vi "Accelerometer.vi"(11 "Queue ref":T1) -> ()   [LabVIEW 2022 SP3]
uses:
  Controls/All Queue.ctl
  Controls/DAQ case.ctl
  Controls/UI Data.ctl
  Controls/All Loop Status.ctl
  <vilib>/DAQmx/read.llb/DAQmx Read (Analog 1D Wfm NChan NSamp).vi
  Create Task/ACC Create Task.vi
  <vilib>/DAQmx/configure/timing.llb/DAQmx Timing (Sample Clock).vi
  Sub VI's/Global 1.vi
  <vilib>/DAQmx/miscellaneous.llb/DAQmx Fill In Error Info.vi
panel:
  # "TC channel list"
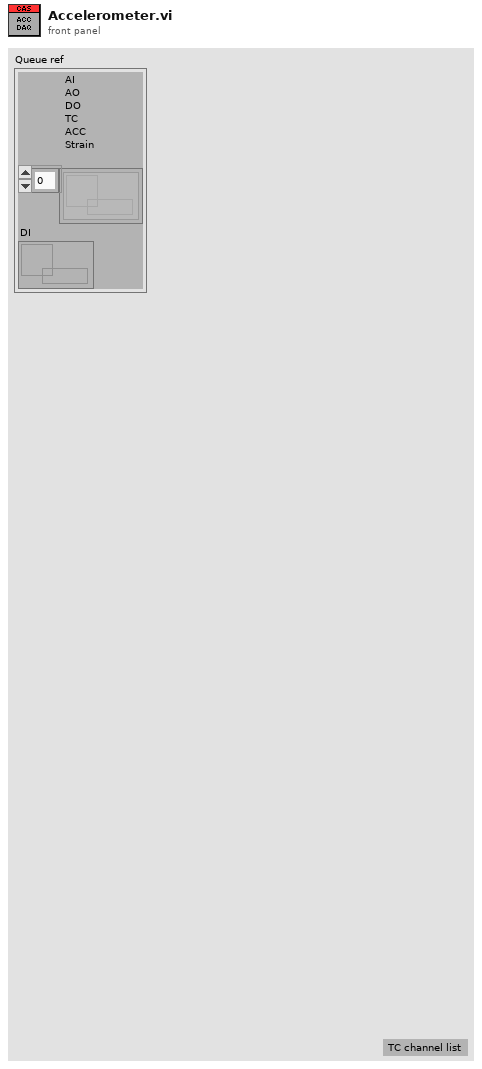
[diagram p1: front panel]
types:
  T1 = typedef "All Queue.ctl" = cluster{"AI\nAO\nDO\nTC\nACC\nStrain":refnum<queue>[], "DI":refnum<queue>}
  T2 = cluster{"in progress?":bool, "Queue ref":T1, "Start DAQ":refnum<notifier>, "UI Data":refnum<notifier>, "task out":refnum<k21>, "ACC Ref":refnum<queue>, "SPC":i32}
  T3 = typedef "DAQ case.ctl" = enum16{"Initailise", "Create Task", "Polevent", "Acquire", "Stop DAQ", "Error", "Exit"}
  T4 = typedef "All Loop Status.ctl" = enum16{"AI", "AO", "DI", "DO", "TC", "Strain", "ACC", "RT", "Log"}
  T5 = enum16{"Init", "Read 'All'", "Read 'n'", "Read '1'", "Write '1'", "Write 'n'", "Write 'All'"}
  T6 = typedef "All Notifer.ctl" = cluster{"UI Data":refnum<notifier>, "Start DAQ":refnum<notifier>, "Start Log":refnum<notifier>}
  T7 = cluster{"Analog input":bool, "Analog Output":bool, "Digital input":bool, "Digital output":bool, "Thermocouple":bool, "Strain Gauge":bool, "Accelerometer":bool}
  T8 = typedef "Config.ctl" = cluster{"AO config":cluster{"Channel_Name":string, "Channel_Number":string, "Default_Value":dbl, "Units":string}[], "AI config":cluster{"Channel_Name":string, "Channel_Number":string, "Pre_Scale_min":dbl, "Pre_Scale_max":dbl, "Sensor_min":dbl, "Sensor_max":dbl, "Units":string}[], "DI config":cluster{"Channel_Name":string, "Channel_Number":string, "Default_Value":bool, "DI invert?":bool}[], "DO config":cluster{"Channel_Name":string, "Channel_Number":string, "Default_Value":bool, "DO invert?":bool}[], "TC config":cluster{"Channel_Name":string, "Channel_Number":string, "Pre_Scale_min":dbl, "Pre_Scale_max":dbl, "units":i32, " type":i32}[], "ACC config":cluster{"Channel_Name":string, "Channel_Number":string, "Pre_Scale_min":dbl, "Pre_Scale_max":dbl, "Terminal configuration":i32, "Sensitivity":dbl, "Sensitivity units":i32}[], "SG config":cluster{"Channel_Name":string, "Channel_Number":string, "Pre_Scale_min":dbl, "Pre_Scale_max":dbl}[], "Strain Gauge Settings":cluster{"poisson ratio":dbl, "nominal gage resistance":dbl, "gage factor":dbl}, "bridge information":cluster{"strain configuration":i32, "lead wire resistance":dbl, "initial bridge voltage":dbl, "voltage excitation source":i32, "voltage excitation value":dbl}, "Sample Rate":cluster{"AI Sample Rate":dbl, "AO Sample Rate":dbl, "DI Sample Rate":dbl, "TC Sample Rate":dbl, "DO Sample Rate":dbl, "SG Sample Rate":dbl, "ACC Sample Rate":dbl}}
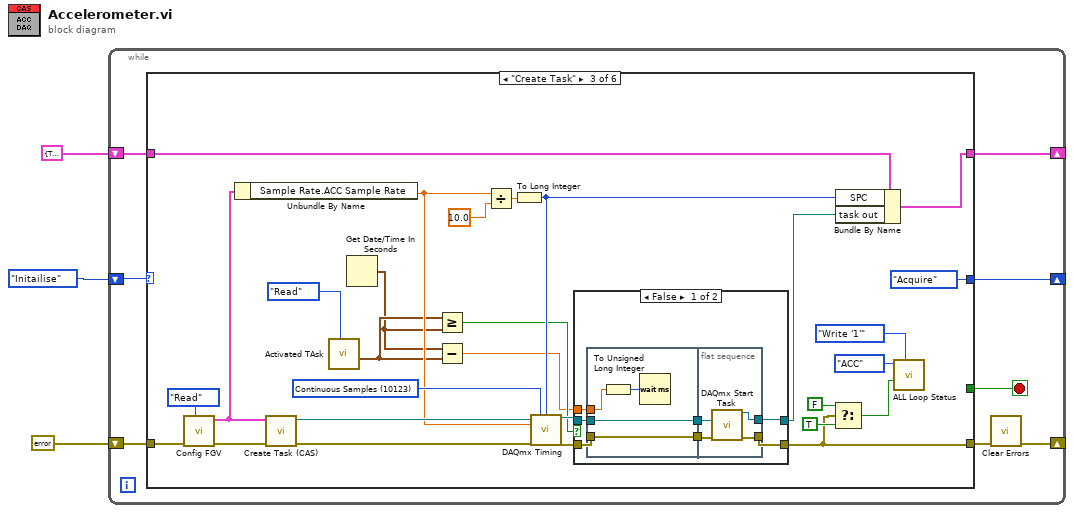
[diagram p0: block diagram]
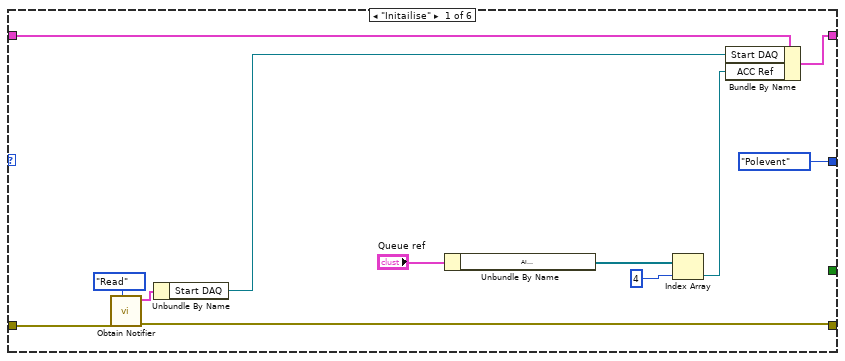
[diagram p2: hidden frame]
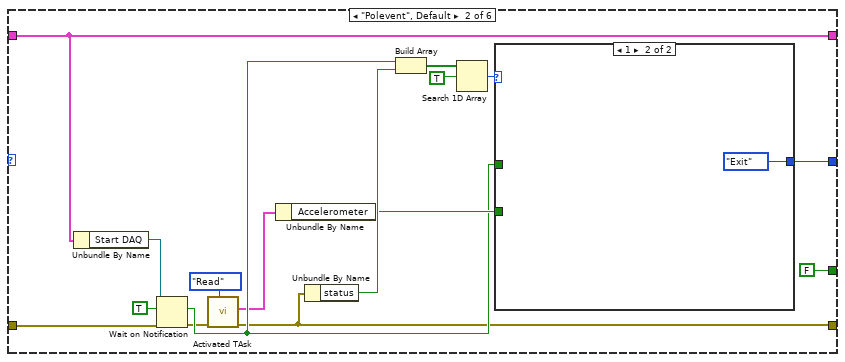
[diagram p3: hidden frame]
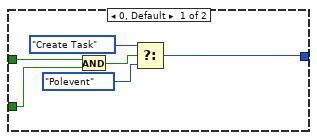
[diagram p4: hidden frame]
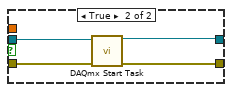
[diagram p5: hidden frame]
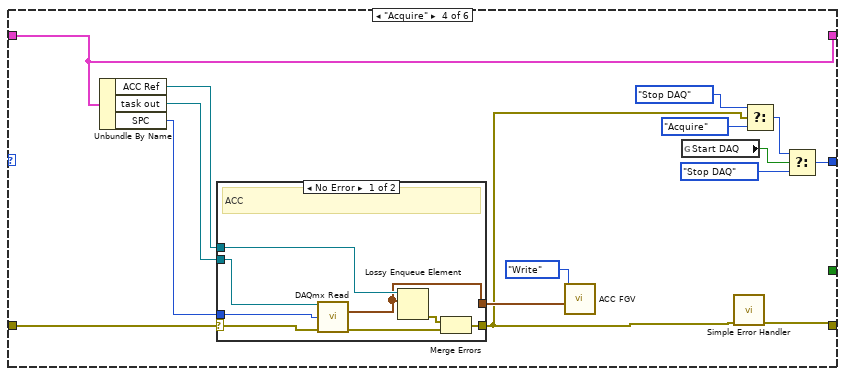
[diagram p6: hidden frame]
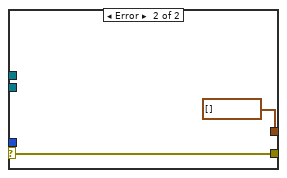
[diagram p7: hidden frame]
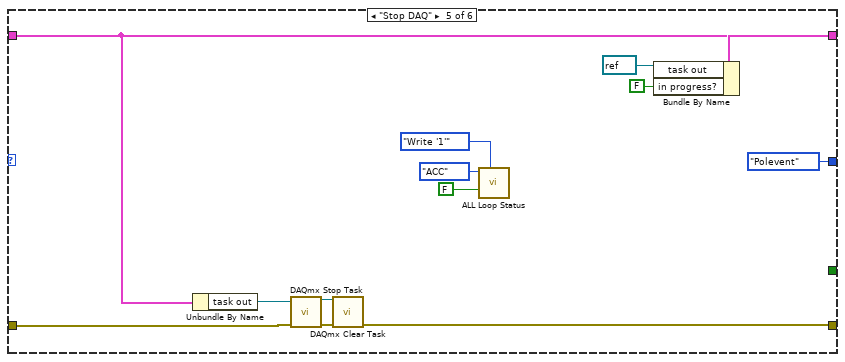
[diagram p8: hidden frame]
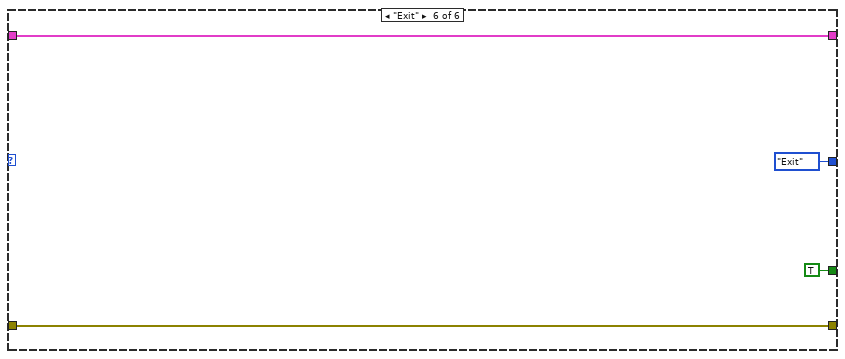
[diagram p9: hidden frame]
diagram:
  n1 = while {
    shift-right: [w4] -> _
    shift-left: errorcluster {"status"=FALSE, "code"=0, "source"=""} ("error out") -> [w10]
    shift-right: [w8] -> _
    shift-left: T2 {"in progress?"=TRUE, "Queue ref"={"AI\nAO\nDO\nTC\nACC\nStrain"=[], "DI"=refnum}, "Start DAQ"=refnum, "UI Data"=refnum, "task out"="", "ACC Ref"=refnum, "SPC"=0} -> [w9]
    shift-right: [w7] -> _
    shift-left: DAQ_case."Initailise" -> [w6]
    stop <- w11 stop-if-true
    n2 = case shown="\"Create Task\"" w6 {
      tunnel: [_ FALSE _ _ _ TRUE] -> w11
      tunnel: w10 -> [w22 w27 w71 w101 w123 w135]
      tunnel: [w21 w25 w54 w95 w124 w135] -> w5
      tunnel: w9 -> [w19 w37 w73 w102 w128 w134]
      tunnel: [w17 w37 w72 w102 w129 w134] -> w8
      tunnel: [DAQ_case."Polevent" w38 DAQ_case."Acquire" w103 DAQ_case."Polevent" DAQ_case."Exit"] -> w7
      frame "Initailise" {
        n3 = call "Obtain Notifier.vi"("Case"=enum16{"Obtain", "Read"}."Read", "error in (no error)"=w22) -> ("error out"=w21:errorcluster, "notifiers out"=w20:T6)  [unwired: 8 in]
        n4 = Unbundle By Name(w20) -> ("Start DAQ"=w18:refnum<notifier>)
        n5 = Unbundle By Name("Queue ref") -> ("AI\nAO\nDO\nTC\nACC\nStrain"=w14:refnum<queue>[])
        n6 = Index Array(array=w14, index=4) -> (element=w13:refnum<queue>)
        n7 = Bundle By Name(cluster=w19, "Start DAQ"=w18, "ACC Ref"=w13) -> (w17:T2)
      }
      frame "Polevent", Default {
        n8 = Unbundle By Name(w37) -> ("Start DAQ"=w36:refnum<notifier>)
        n9 = Wait on Notification(notifier=w36, ignore previous (F)=TRUE, error in (no error)=w27) -> (notification=w28:bool, error out=w26:errorcluster)  [unwired: 1 in, 2 out]
        n10 = call "Activated TAsk.vi"("Enum"=enum16{"Read", "Write"}."Read", "error in (no error)"=w26) -> ("error out"=w25:errorcluster, "Activate Task 2"=w24:T7)  [unwired: 7 in, 1 out]
        n11 = Unbundle By Name(w24) -> ("Accelerometer"=w29:bool)
        n12 = Unbundle By Name(w25) -> ("status"=w35:bool)
        n13 = Build Array(w28, w35) -> (w33:bool[])
        n14 = Search 1D Array(1D array=w33, element=TRUE) -> (index of element=w31:i32)  [unwired: 1 in]
        n15 = case shown="1" w31 {
          tunnel: [w44 DAQ_case."Exit"] -> w38
          tunnel: w29 -> [w41 _]
          tunnel: w28 -> [w40 _]
          frame 0, Default {
            n16 = And(x=w40, y=w41) -> (x .and. y?=w42:bool)
            n17 = Select(t=DAQ_case."Create Task", s=w42, f=DAQ_case."Polevent") -> (s? t:f=w44:T3)
          }
          frame 1 {
          }
        }
      }
      frame "Create Task" {
        w65 = 10123 items=["Finite Samples"=10178, "Continuous Samples"=10123, "Hardware Timed Single Point"=12522] ("sample mode")
        n18 = call "Config FGV.vi"("Enum"=enum16{"Read", "Write"}."Read", "error in (no error)"=w71) -> ("error out"=w68:errorcluster, "Data"=w59:T8)  [unwired: 8 in]
        n19 = Unbundle By Name(w59) -> ("Sample Rate.ACC Sample Rate"=w56:dbl)
        n20 = call-poly "Create Task (CAS).vi"("error in"=w68, "Config"=w59) -> ("error out"=w66:errorcluster, "ACC Task"=w67:refnum<k21>)  [unwired: 8 in]
        n21 = call "Activated TAsk.vi"("Enum"=enum16{"Read", "Write"}."Read") -> ("Start Time"=w48:timestamp)  [unwired: 8 in, 2 out]
        n22 = Get Date/Time In Seconds() -> (seconds since 1Jan1904=w47:timestamp)
        n23 = Greater Or Equal?(x=w48, y=w47) -> (x >= y?=w51:bool)
        n24 = Subtract(x=w47, y=w48) -> (x-y=w50:dbl)
        n25 = Divide(x=w56, y=10.0) -> (x/y=w57:dbl)
        n26 = To Long Integer(number=w57) -> (32bit integer=w55:i32)
        n27 = call-poly <vilib>:"DAQmx Timing.vi"("task/channels in"=w67, "sample mode"=w65, "samples per channel"=w55, "rate"=w56, "error in"=w66) -> ("task out"=w52:refnum<k21>, "error out"=w53:errorcluster)  [unwired: 9 in]
        n28 = case shown="False" w51 {
          tunnel: w53 -> [w81 w93]
          tunnel: [w80 w92] -> w54
          tunnel: w52 -> [w79 w90]
          tunnel: [w78 w91] -> w49
          tunnel: w50 -> [w75 _]
          frame False {
            n29 = flat-sequence {
              tunnel: w79 -> [w84]
              tunnel: w81 -> [w85]
              tunnel: [w85] -> w77
              tunnel: [w84] -> w76
              tunnel: w75 -> [w82]
              tunnel: [w88] -> w80
              tunnel: [w86] -> w78
              tunnel: w77 -> [w89]
              tunnel: w76 -> [w87]
              frame #0 {
                n30 = To Unsigned Long Integer(number=w82) -> (unsigned 32bit integer=w83:u32)
                n31 = Wait (ms)(milliseconds to wait=w83) -> ()  [unwired: 1 out]
              }
              frame #1 {
                n32 = call <vilib>:"DAQmx Start Task.vi"("task/channels in"=w87, "error in"=w89) -> ("task out"=w86:refnum<k21>, "error out"=w88:errorcluster)  [unwired: 12 in]
              }
            }
          }
          frame True {
            n33 = call <vilib>:"DAQmx Start Task.vi"("task/channels in"=w90, "error in"=w93) -> ("task out"=w91:refnum<k21>, "error out"=w92:errorcluster)  [unwired: 12 in]
          }
        }
        n34 = Select(t=FALSE, s=w54, f=TRUE) -> (s? t:f=w62:bool)
        n35 = Bundle By Name(cluster=w73, "SPC"=w55, "task out"=w49) -> (w72:T2)
        n36 = call "ALL Loop Status.vi"("Option"=T5."Write '1'", "Status"=w62, "Loop"=All_Loop_Status."ACC") -> ()  [unwired: 6 in, 3 out]
      }
      frame "Acquire" {
        n37 = Unbundle By Name(w102) -> ("ACC Ref"=w100:refnum<queue>, "task out"=w99:refnum<k21>, "SPC"=w94:i32)
        n38 = case shown="No Error" w101 {
          selector: w101 -> [w112 w118]
          tunnel: w99 -> [w111 _]
          tunnel: [w114 w118] -> w96
          tunnel: w100 -> [w113 _]
          tunnel: [w110 waveform(dbl)[] [] ("data")] -> w98
          tunnel: w94 -> [w109 _]
          frame No Error {
            # "ACC"
            n39 = call-poly <vilib>:"DAQmx Read.vi"("task/channels in"=w111, "number of samples per channel"=w109, "error in"=w112) -> ("data"=w110:waveform(dbl)[], "error out"=w115:errorcluster)  [unwired: 10 in, 1 out]
            n40 = Lossy Enqueue Element(queue=w113, element=w110) -> (error out=w116:errorcluster)  [unwired: 1 in, 3 out]
            n41 = Merge Errors(w116, w115) -> (w114:errorcluster)
          }
          frame Error {
          }
        }
        n42 = call "ACC FGV.vi"("AI data"=w98, "Enum"=enum16{"Read", "Write"}."Write") -> ()  [unwired: 9 in, 1 out]
        n43 = global read "Global 1.vi" "Start DAQ"() -> (w106:bool)
        n44 = call <vilib>:"Simple Error Handler.vi"("error in (no error)"=w96) -> ("error out"=w95:errorcluster)  [unwired: 4 in, 4 out]
        n45 = Select(t=DAQ_case."Stop DAQ", s=w96, f=DAQ_case."Acquire") -> (s? t:f=w105:T3)
        n46 = Select(t=w105, s=w106, f=DAQ_case."Stop DAQ") -> (s? t:f=w103:T3)
      }
      frame "Stop DAQ" {
        n47 = Unbundle By Name(w128) -> ("task out"=w122:refnum<k21>)
        n48 = call <vilib>:"DAQmx Stop Task.vi"("task/channels in"=w122, "error in"=w123) -> ("task out"=w121:refnum<k21>, "error out"=w125:errorcluster)  [unwired: 12 in]
        n49 = call <vilib>:"DAQmx Clear Task.vi"("task in"=w121, "error in"=w125) -> ("error out"=w124:errorcluster)  [unwired: 13 in]
        n50 = call "ALL Loop Status.vi"("Option"=T5."Write '1'", "Status"=FALSE, "Loop"=All_Loop_Status."ACC") -> ()  [unwired: 6 in, 3 out]
        n51 = Bundle By Name(cluster=w128, "task out"=refnum<k21> refnum, "in progress?"=FALSE) -> (w129:T2)
      }
      frame "Exit" {
      }
    }
    n52 = call <vilib>:"Clear Errors.vi"("error in (no error)"=w5) -> ("error out"=w4:errorcluster)  [unwired: 5 in, 1 out]
  }
